vi "Create Plugin Groups.vi"(8 "error in (no error)":errorcluster, 9 "String":string, 10 "dsf refnum in":refnum<class "Configuration Session.lvclass">, 11 "Section Ptr":T1 format="%.0x") -> (0 "error out":errorcluster)   [LabVIEW 2017, in "DSF System Explorer.lvlib"]
uses:
  DSF System Explorer.lvlib
  <vilib>/NI Veristand/Custom Device API/Custom Device Item Ref.ctl
  DSF Core.lvlibp/Classes/Configuration/Configuration Session.lvclass
  DSF Core.lvlibp/Classes/Configuration/Read Plugin Group IDs.vi
  DSF Core.lvlibp/Classes/Configuration/Read Group.vi
  <vilib>/NI Veristand/Custom Device API/Custom Device API.lvlib
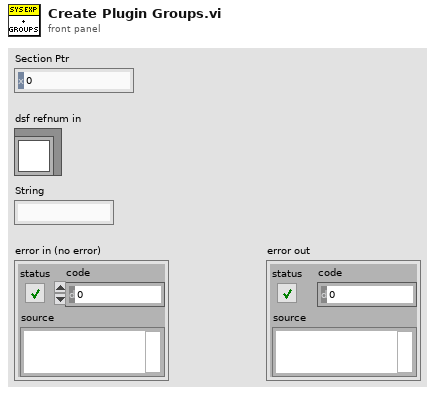
[diagram p1: front panel]
types:
  T1 = typedef "Custom Device API.lvlib/Custom Device Item Ref.ctl" = u64
  T2 = typedef "DSF Core.lvlibp/DSF Group Info.ctl" = cluster{"direction":T3, "timing":T4, "transfer ids":string[], "settings id":string, "thread":i32, "timeout behavior":T5}
  T3 = typedef "DSF Core.lvlibp/DSF Direction.ctl" = enum8{"Tx", "Rx"}
  T4 = typedef "DSF Core.lvlibp/DSF Timing Info.ctl" = cluster{"priority":u64, "decimation":u64, "offset":u64}
  T5 = typedef "DSF Core.lvlibp/DSF Timeout Behavior.ctl" = enum8{"Increment Late Count", "Throw Error"}
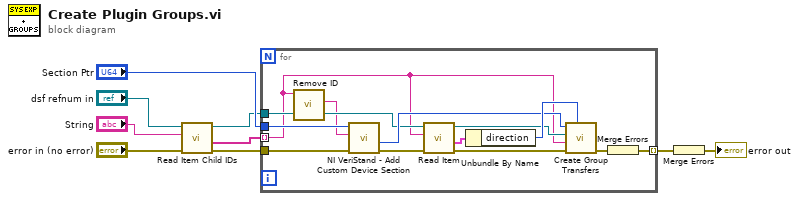
[diagram p0: block diagram]
diagram:
  n1 = call-poly "Read Item Child IDs.vi"("error in (no error)"="error in (no error)", "Plugin ID"="String", "Configuration Session"="dsf refnum in") -> ("error out"=w4:errorcluster, "Group IDs"=w3:string[], "Configuration Session out"=w2:refnum<class "Configuration Session.lvclass">)  [unwired: 5 in, 1 out]
  n2 = for {
    tunnel: w3 -> [w10] mode=indexing
    tunnel: "Section Ptr" -> [w22]
    tunnel: w4 -> [w21]
    tunnel: [w20] -> w8 mode=indexing
    tunnel: w2 -> [w16]
    n3 = call "Remove ID.vi"("id string"=w10) -> ("name"=w11:string)  [unwired: 9 in, 1 out]
    n4 = call <vilib>:"NI VeriStand - Add Custom Device Section.vi"("error in (no error)"=w21, "Section Name"=w11, "Parent Ref in"=w22) -> ("error out"=w15:errorcluster, "Section Ptr"=w17:T1)  [unwired: 5 in, 2 out]
    n5 = call-poly "Read Item.vi"("error in (no error)"=w15, "Group ID"=w10, "Configuration Session in"=w16) -> ("error out"=w13:errorcluster, "value"=w12:T2, "Configuration Session out"=w14:refnum<class "Configuration Session.lvclass">)  [unwired: 5 in, 1 out]
    n6 = Unbundle By Name(w12) -> ("direction"=w19:T3)
    n7 = call "Create Group Transfers.vi"("direction"=w19, "error in (no error)"=w13, "Group ID"=w10, "dsf refnum in"=w14, "Section Ptr"=w17) -> ("error out"=w18:errorcluster)  [unwired: 6 in]
    n8 = Merge Errors(w18) -> (w20:errorcluster)
  }
  n9 = Merge Errors(w8) -> (→"error out":errorcluster)
